vi "SetIFTrackSwitchSts.vi"(8 "错误输入（无错误）":errorcluster, 10 "闸门跟踪属性":i32) -> (0 "错误输出":errorcluster)   [LabVIEW 2014]
uses:
  X86Dll/ZXUTConfigMgr.dll
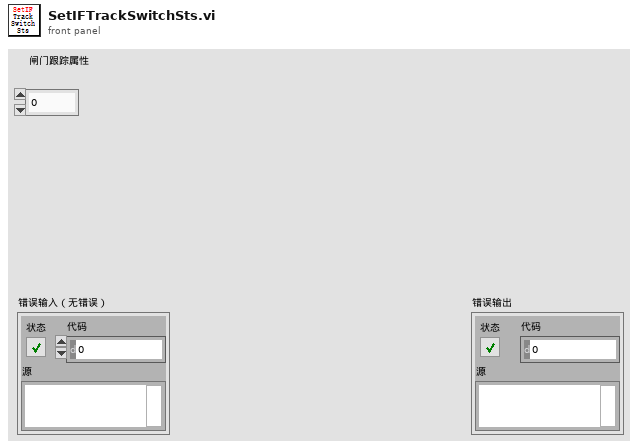
[diagram p1: front panel]
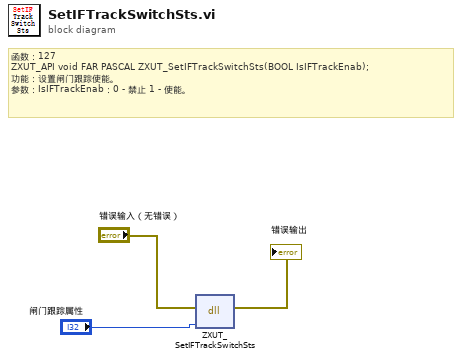
[diagram p0: block diagram]
diagram:
  # "函数：127\nZXUT_API void\tFAR PASCAL ZXUT_SetIFTrackSwitchSts(BOOL IsIFTrackEnab);\n功能：设置闸门跟踪使能。\n参数：IsIFTrackEnab：0 - 禁止 1 - 使能。"
  n1 = dll-call lib="D:/Software/Utrasonic on-line monitoring/X86Dll/ZXUTConfigMgr.dll" fn="ZXUT_SetIFTrackSwitchSts"(error in="错误输入（无错误）", "IsIFTrackEnab"="闸门跟踪属性") -> (error out=→"错误输出":errorcluster)  [unwired: 4 in, 1 out]
